vi "Configure Delay.vi"(8 "error in (no error)":errorcluster, 10 "Set Delay (0 s)":dbl format="%.2f", 11 "VISA resource name":refnum<visa-resource-name>) -> (0 "error out":errorcluster, 3 "VISA resource name out":refnum<visa-resource-name>)   [LabVIEW 2021, in "Sorensen M9A Series.lvlib"]
doc: "This VI sets the delay before reporting fault conditions after a new output setting is specified for the Sorensen power supply. Units are in seconds."
uses:
  Sorensen M9A Series.lvlib
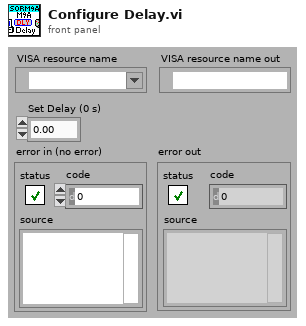
[diagram p1: front panel]
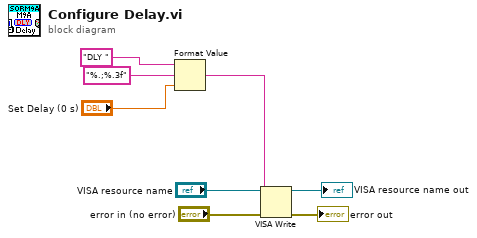
[diagram p0: block diagram]
diagram:
  n1 = Format Value(string ("")="DLY " ("data"), format string="%.;%.3f", value (0)="Set Delay (0 s)") -> (output string=w4:string)
  n2 = VISA Write(VISA resource name="VISA resource name", write buffer=w4, error in (no error)="error in (no error)") -> (VISA resource name out=→"VISA resource name out":refnum<visa-resource-name>, error out=→"error out":errorcluster)  [unwired: 1 out]
